vi "PH_Beckhoff_PP_PU.handle HV Meas.vi"(0 "i ref in":refnum<vi>, 4 "Values":T2, 5 "error in":errorcluster, 7 "Values changed at":T1) -> (14 "i ref out":refnum<vi>, 19 "error out":errorcluster)   [LabVIEW 2014, in "PH_Beckhoff_PP_PU.lvlib"]
doc: "This VI handles the incoming information about HV Meas inputs: If the value* or quality changed, these are set to own attributes and the scaled information is published via DIM.\n\n*: in this case a value change means that the calculated voltage changed by one or more steps in multiples of 100V of the calculated voltage."
uses:
  PH_Beckhoff_PP_PU.lvlib
  PH_Beckhoff/PH_Beckhoff.Values.ctl
  PH_Beckhoff/PH_Beckhoff.Sonderklemmen Inputs.ctl
  PH_Beckhoff/PH_Beckhoff.Analog Inputs.ctl
  PH_Beckhoff/PH_Beckhoff.Scaling Type.ctl
  PH_Beckhoff/PH_Beckhoff.Analog Outputs.ctl
  PH_Beckhoff/PH_Beckhoff.Digital Inputs.ctl
  PH_Beckhoff/PH_Beckhoff.Digital Outputs.ctl
  PH_Beckhoff/PH_Beckhoff.lvlib
  PH_Common/PH_Common.lvlib
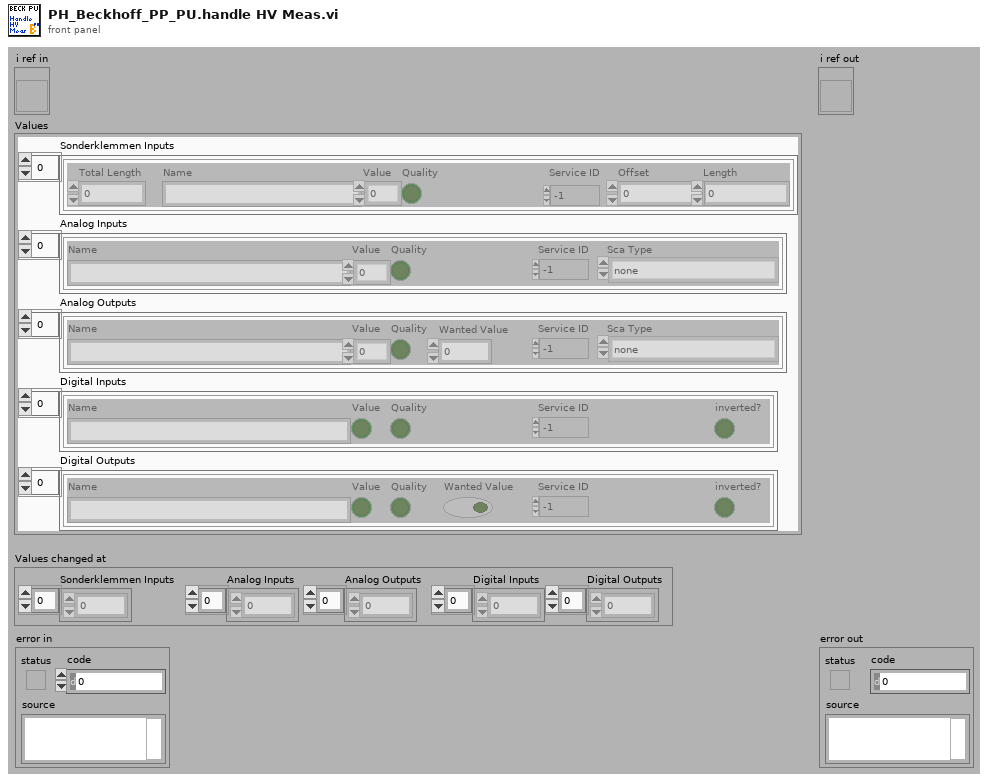
[diagram p1: front panel]
types:
  T1 = cluster{"Sonderklemmen Inputs":i32[], "Analog Inputs":i32[], "Analog Outputs":i32[], "Digital Inputs":i32[], "Digital Outputs":i32[]}
  T2 = typedef "PH_Beckhoff.lvlib/PH_Beckhoff.Values.ctl" = cluster{"Sonderklemmen Inputs":T3, "Analog Inputs":T4, "Analog Outputs":T6, "Digital Inputs":T7, "Digital Outputs":T8}
  T3 = typedef "PH_Beckhoff.lvlib/PH_Beckhoff.Sonderklemmen Inputs.ctl" = cluster{"Total Length":u32, "Name":string, "Value":u64, "Quality":bool, "Service ID":i32, "Offset":u32, "Length":u32}[]
  T4 = typedef "PH_Beckhoff.lvlib/PH_Beckhoff.Analog Inputs.ctl" = cluster{"Name":string, "Value":u32, "Quality":bool, "Service ID":i32, "Sca Type":T5}[]
  T5 = typedef "PH_Beckhoff.lvlib/PH_Beckhoff.Scaling Type.ctl" = enum16{"none", "0 ... 15 Bit -> 0 ... 5", "0 ... 15 Bit -> 0 ... 10", "0 ... 15 Bit -> 0 ... 25", "0 ... 15 Bit -> 4 ... 20", "0 ... 15 Bit -> 0 ... 1", "0 ... 15 Bit -> 0 ... 20000", "0 ... 15 Bit -> 0 ... 24000"}
  T6 = typedef "PH_Beckhoff.lvlib/PH_Beckhoff.Analog Outputs.ctl" = cluster{"Name":string, "Value":u32, "Quality":bool, "Wanted Value":u32, "Service ID":i32, "Sca Type":T5}[]
  T7 = typedef "PH_Beckhoff.lvlib/PH_Beckhoff.Digital Inputs.ctl" = cluster{"Name":string, "Value":bool, "Quality":bool, "Service ID":i32, "inverted?":bool}[]
  T8 = typedef "PH_Beckhoff.lvlib/PH_Beckhoff.Digital Outputs.ctl" = cluster{"Name":string, "Value":bool, "Quality":bool, "Wanted Value":bool, "Service ID":i32, "inverted?":bool}[]
  T9 = typedef "PH_Beckhoff_PP_PU.lvlib/PH_Beckhoff_PP_PU.i attribute.ctl" = cluster{"HV Meas":cluster{"Input GUI Ref":refnum<vi>, "Voltage Service ID":i32, "Voltage [V]":dbl, "Quality":bool, "# in Data":i32}[], "Trigger":cluster{"Status":cluster{"GUI Ref":refnum<vi>, "Status Service ID":i32, "Status":T10}, "last shot:":cluster{"GUI Ref":refnum<vi>, "Service ID":i32, "Time":string}, "DIs":cluster{"triggered":cluster{"GUI Ref":refnum<vi>, "# in Data":i32}, "fired":cluster{"GUI Ref":refnum<vi>, "# in Data":i32}}, "GUI Ref Indicator":refnum<vi>}[], "RR":cluster{"Status":cluster{"GUI Ref":refnum<vi>, "Status Service ID":i32, "Status":T10}, "DIs":cluster{"closed":cluster{"GUI Ref":refnum<vi>, "# in Data":i32}, "open":cluster{"GUI Ref":refnum<vi>, "# in Data":i32}}, "Close":cluster{"GUI Ref":refnum<vi>, "# in Data":i32}, "GUI Ref Indicator":refnum<vi>}[], "Igni":cluster{"Status":cluster{"GUI Ref":refnum<vi>, "Status Service ID":i32, "Status":T10}, "DIs":cluster{"heating on":cluster{"GUI Ref":refnum<vi>, "# in Data":i32}, "water on":cluster{"GUI Ref":refnum<vi>, "# in Data":i32}}, "Device on":cluster{"GUI Ref":refnum<vi>, "# in Data":i32}, "GUI Ref Indicator":refnum<vi>}[], "PSU":cluster{"Status":cluster{"GUI Ref":refnum<vi>, "Status Service ID":i32, "Status":T10}, "Limit Service ID":i32, "DIs":cluster{"inhibit":cluster{"GUI Ref":refnum<vi>, "# in Data":i32}, "end of charge":cluster{"GUI Ref":refnum<vi>, "# in Data":i32}, "HV on":cluster{"GUI Ref":refnum<vi>, "# in Data":i32}, "overtemp":cluster{"GUI Ref":refnum<vi>, "# in Data":i32}, "interlock":cluster{"GUI Ref":refnum<vi>, "# in Data":i32}, "load fault":cluster{"GUI Ref":refnum<vi>, "# in Data":i32}, "sum fault":cluster{"GUI Ref":refnum<vi>, "# in Data":i32}, "HV off":cluster{"GUI Ref":refnum<vi>, "# in Data":i32}, "DC ok":cluster{"GUI Ref":refnum<vi>, "# in Data":i32}}, "AIs":cluster{"voltage":cluster{"GUI Ref":refnum<vi>, "# in Data":i32}, "current":cluster{"GUI Ref":refnum<vi>, "# in Data":i32}}, "DAs":cluster{"inhibit":cluster{"GUI Ref":refnum<vi>, "# in Data":i32}, "interlock":cluster{"GUI Ref":refnum<vi>, "# in Data":i32}, "HV on":cluster{"GUI Ref":refnum<vi>, "# in Data":i32}, "Reset":cluster{"GUI Ref":refnum<vi>, "# in Data":i32}}, "AAs":cluster{"Voltage to set":cluster{"GUI Ref":refnum<vi>, "# in Data":i32}}, "GUI Ref Indicator":refnum<vi>}[], "reconfigured":cluster{"?":bool, "GUI Ref":refnum<vi>}, "PU Rack Type":T11, "HV Meas Info":T12, "PSU Info":T13}
  T10 = typedef "PH_StatusHandler.lvlib/PH_StatusHandler.Status.ctl" = i16
  T11 = typedef "PH_Beckhoff_PP_PU.lvlib/PH_Beckhoff_PP_PU.PU Rack Type.ctl" = enum16{"no Info", "PA 19mm", "PA 45mm", "MA PU 1 and 2", "MA PU 3 and 4", "MA PU 5 and 6", "MA FR and PILC"}
  T12 = typedef "PH_Beckhoff_PP_PU.lvlib/PH_Beckhoff_PP_PU.HV Meas Info.ctl" = cluster{"Period Time [s]":dbl, "Subtractor 1 [Hz]":dbl, "Devider 1 [Hz/kV]":dbl, "Subtractor 2 [Hz]":dbl, "Devider 2 [Hz/kV]":dbl}
  T13 = typedef "PH_Beckhoff_PP_PU.lvlib/PH_Beckhoff_PP_PU.PSU Info.ctl" = cluster{"Limits 1 [V]":cluster{"Lower":dbl, "Upper":dbl}, "Limits 2 [V]":cluster{"Lower":dbl, "Upper":dbl}}
  T14 = cluster{"Input GUI Ref":refnum<vi>, "Voltage Service ID":i32, "Voltage [V]":dbl, "Quality":bool, "# in Data":i32}[]
  T15 = cluster{"Input GUI Ref":refnum<vi>, "Voltage Service ID":i32, "Voltage [V]":dbl, "Quality":bool, "# in Data":i32}
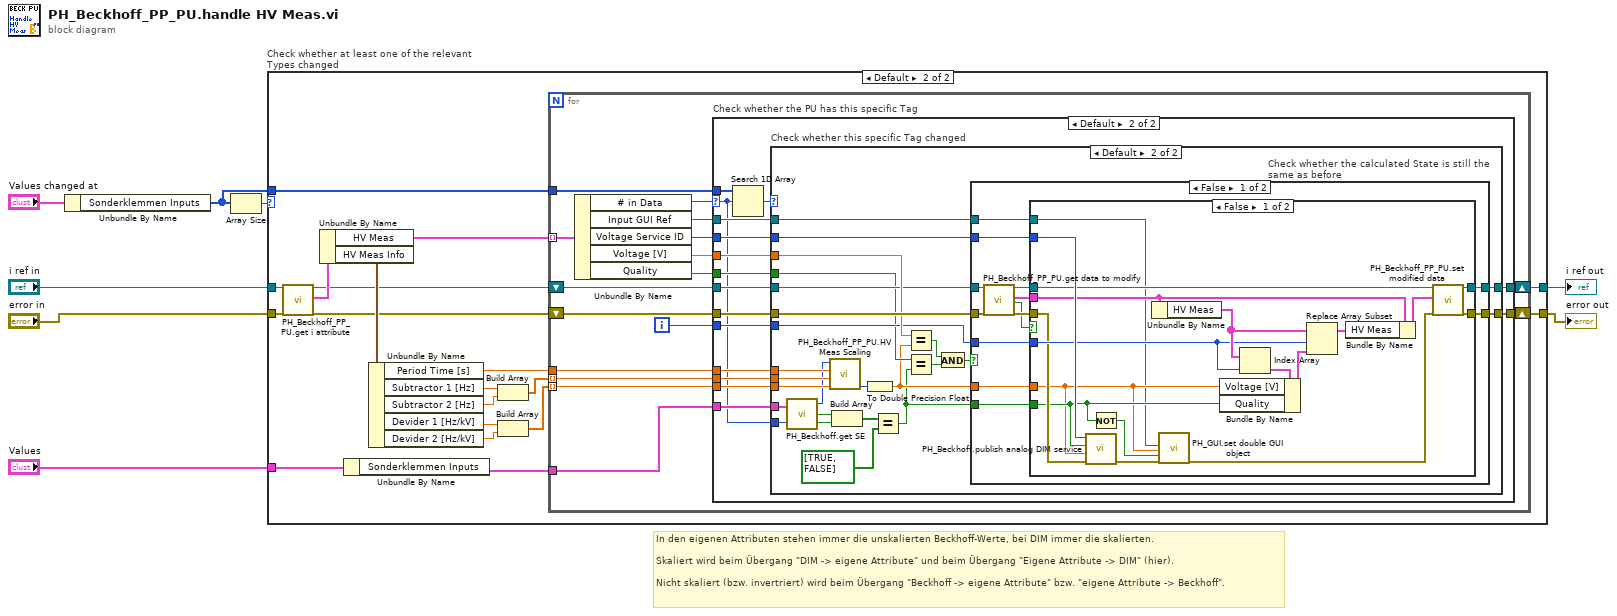
[diagram p0: block diagram]
diagram:
  # "In den eigenen Attributen stehen immer die unskalierten Beckhoff-Werte, bei DIM immer die skalierten.\n\nSkaliert wird beim Übergang \"DIM -> eigene Attribute\" und beim Übergang \"Eigene Attribute -> DIM\" (hier).\n\nNicht skaliert (bzw. invertriert) wird beim Übergang \"Beckhoff -> eigene Attribute\" bzw. \"eigene Attribute -> Beckhoff\"."
  n1 = Unbundle By Name("Values changed at") -> ("Sonderklemmen Inputs"=w3:i32[])
  n2 = Array Size(array=w3) -> (size(s)=w4:i32)
  n3 = case "Check whether at least one of the relevant Types changed" shown="Default" w4 {
    tunnel: [w9 w29] -> w8
    tunnel: [w10 w26] -> w7
    tunnel: "Values" -> [_ w19]
    tunnel: "i ref in" -> [w10 w17]
    tunnel: "error in" -> [w9 w18]
    tunnel: w3 -> [_ w14]
    frame 0 {
    }
    frame Default {
      n4 = call "PH_Beckhoff_PP_PU.get i attribute.vi"("i ref in"=w17, "error in (no error)"=w18) -> ("i ref out"=w12:refnum<vi>, "i attribute"=w16:T9, "error out"=w11:errorcluster)  [unwired: 15 in]
      n5 = Unbundle By Name(w16) -> ("HV Meas"=w15:T14, "HV Meas Info"=w13:T12)
      n6 = Unbundle By Name(w19) -> ("Sonderklemmen Inputs"=w20:T3)
      n7 = Unbundle By Name(w13) -> ("Period Time [s]"=w25:dbl, "Subtractor 1 [Hz]"=w24:dbl, "Subtractor 2 [Hz]"=w23:dbl, "Devider 1 [Hz/kV]"=w22:dbl, "Devider 2 [Hz/kV]"=w21:dbl)
      n8 = Build Array(w24, w23) -> (w28:dbl[])
      n9 = Build Array(w22, w21) -> (w27:dbl[])
      n10 = for "This class is supposed to handle 2 Sonderklemmen of Type KL 5111" {
        shift-right: [w32] -> w29
        shift-left: w11 -> [w40]
        tunnel: w28 -> [w44] mode=indexing
        tunnel: w27 -> [w43] mode=indexing
        tunnel: w25 -> [w45]
        tunnel: w15 -> [w42] mode=indexing
        shift-right: [w37] -> w26
        shift-left: w12 -> [w38]
        tunnel: w20 -> [w34]
        tunnel: w14 -> [w31]
        i -> [w36]
        n11 = Unbundle By Name(w42) -> ("# in Data"=w30:i32, "Input GUI Ref"=w33:refnum<vi>, "Voltage Service ID"=w41:i32, "Voltage [V]"=w39:dbl, "Quality"=w35:bool)
        n12 = case "Check whether the PU has this specific Tag" shown="Default" w30 {
          selector: w30 -> [_ w48]
          tunnel: w45 -> [_ w63]
          tunnel: w44 -> [_ w62]
          tunnel: w43 -> [_ w61]
          tunnel: w41 -> [_ w60]
          tunnel: w40 -> [w47 w59]
          tunnel: w39 -> [_ w58]
          tunnel: w38 -> [w46 w57]
          tunnel: [w46 w56] -> w37
          tunnel: w36 -> [_ w55]
          tunnel: w35 -> [_ w54]
          tunnel: w34 -> [_ w53]
          tunnel: w33 -> [_ w52]
          tunnel: [w47 w51] -> w32
          tunnel: w31 -> [_ w50]
          frame -1 {
          }
          frame Default {
            n13 = Search 1D Array(1D array=w50, element=w48) -> (index of element=w49:i32)  [unwired: 1 in]
            n14 = case "Check whether this specific Tag changed" shown="Default" w49 {
              tunnel: w63 -> [_ w90]
              tunnel: w62 -> [_ w89]
              tunnel: w61 -> [_ w88]
              tunnel: w60 -> [_ w86]
              tunnel: w59 -> [w64 w85]
              tunnel: w58 -> [_ w84]
              tunnel: w57 -> [w65 w82]
              tunnel: [w65 w81] -> w56
              tunnel: w55 -> [_ w80]
              tunnel: w54 -> [_ w79]
              tunnel: w53 -> [_ w76]
              tunnel: w52 -> [_ w66]
              tunnel: [w64 w67] -> w51
              tunnel: w48 -> [_ w68]
              frame -1 {
              }
              frame Default {
                n15 = call "PH_Beckhoff.get SE.vi"("Sonderklemmen Inputs"=w76, "index of element"=w68) -> ("DIM value"=w71:u32, "Quality"=w70:bool, "Tag not found"=w69:bool)
                n16 = call "PH_Beckhoff_PP_PU.HV Meas Scaling.vi"("Devider [Hz/kV]"=w88, "Subtractor [Hz]"=w89, "Period Time [s]"=w90, "Beckhoff value"=w71) -> ("Spannung [V]"=w87:i32)  [unwired: 3 in]
                n17 = Build Array(w70, w69) -> (w75:bool[])
                n18 = To Double Precision Float(number=w87) -> (double precision float=w73:dbl)
                n19 = Equal?(x=w75, y=bool[] [TRUE, FALSE] ("appended array")) -> (x = y?=w72:bool)
                n20 = Equal?(x=w84, y=w73) -> (x = y?=w83:bool)
                n21 = Equal?(x=w79, y=w72) -> (x = y?=w77:bool)
                n22 = And(x=w83, y=w77) -> (x .and. y?=w78:bool)
                n23 = case "Check whether the calculated State is still the same as before" shown="False" w78 {
                  tunnel: [w98 w124] -> w67
                  tunnel: w72 -> [w92 _]
                  tunnel: w86 -> [w103 _]
                  tunnel: w85 -> [w102 w124]
                  tunnel: w73 -> [w101 _]
                  tunnel: w82 -> [w99 w125]
                  tunnel: [w96 w125] -> w81
                  tunnel: w80 -> [w94 _]
                  tunnel: w66 -> [w91 _]
                  frame False {
                    n24 = call "PH_Beckhoff_PP_PU.get data to modify.vi"("i ref in"=w99, "error in (no error)"=w102) -> ("i ref out"=w97:refnum<vi>, "i attribute"=w95:T9, "timed out"=w93:bool, "error out"=w100:errorcluster)  [unwired: 14 in]
                    n25 = case shown="False" w93 {
                      tunnel: w92 -> [w106 _]
                      tunnel: w103 -> [w121 _]
                      tunnel: w101 -> [w105 _]
                      tunnel: w100 -> [w110 w122]
                      tunnel: [w120 w122] -> w98
                      tunnel: w97 -> [w119 w123]
                      tunnel: [w118 w123] -> w96
                      tunnel: w95 -> [w117 _]
                      tunnel: w94 -> [w113 _]
                      tunnel: w91 -> [w104 _]
                      frame False {
                        n26 = call "PH_Beckhoff.publish analog DIM service.vi"("error in"=w110, "Value"=w105, "Quality ok?"=w106, "Service ID"=w121) -> ("error out"=w109:errorcluster)  [unwired: 4 in]
                        n27 = Not(x=w106) -> (.not. x?=w107:bool)
                        n28 = Unbundle By Name(w117) -> ("HV Meas"=w114:T14)
                        n29 = call "PH_GUI.set double GUI object.vi"("GUI object Ref"=w104, "value"=w105, "blinking (false)"=w107, "error in (no error)"=w109) -> ("error out"=w108:errorcluster)  [unwired: 15 in]
                        n30 = Index Array(array=w114, index=w113) -> (element=w112:T15)
                        n31 = Bundle By Name(cluster=w112, "Voltage [V]"=w105, "Quality"=w106) -> (w111:T15)
                        n32 = Replace Array Subset(array=w114, new element=w111, index=w113) -> (w115:T14)
                        n33 = Bundle By Name(cluster=w117, "HV Meas"=w115) -> (w116:T9)
                        n34 = call "PH_Beckhoff_PP_PU.set modified data.vi"("i ref in"=w119, "i attribute"=w116, "error in (no error)"=w108) -> ("i ref out"=w118:refnum<vi>, "error out"=w120:errorcluster)  [unwired: 15 in]
                      }
                      frame True {
                      }
                    }
                  }
                  frame True {
                  }
                }
              }
            }
          }
        }
      }
    }
  }
  "i ref out" <- w7
  "error out" <- w8
